vi "Result Response.vi"(8 "error in (no error)":errorcluster, 10 "Acquired Result.lvclass":refnum<class "Acquired Result.lvclass">, 11 "Measure Controller in":refnum<class "Measure Controller.lvclass">) -> (0 "error out":errorcluster, 3 "Measure Controller out":refnum<class "Measure Controller.lvclass">)   [LabVIEW 2015, in "Measure Controller.lvclass"]
uses:
  Measure Controller.lvclass
  Results/Acquired Result/Acquired Result.lvclass
  Measure Object/Measure Object.lvclass/Measure Object.ctl
  Measure Object/Read tdms stream.vi
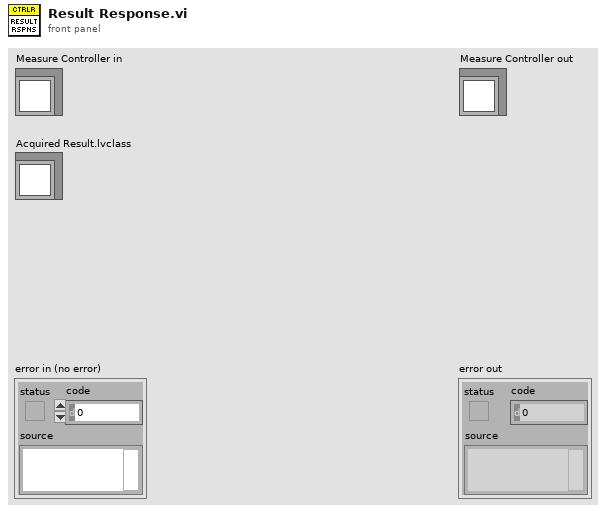
[diagram p1: front panel]
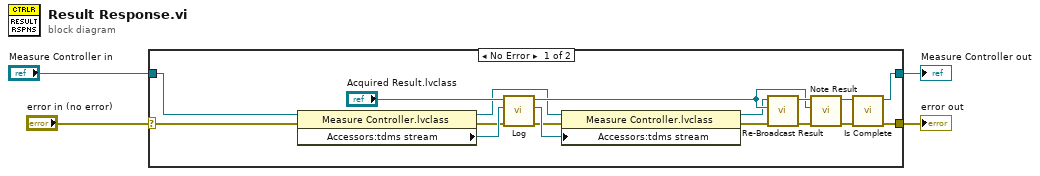
[diagram p0: block diagram]
diagram:
  n1 = case shown="No Error" "error in (no error)" {
    selector: "error in (no error)" -> [w10 w23]
    tunnel: [w20 w23] -> w3
    tunnel: [w21 w22] -> w1
    tunnel: "Measure Controller in" -> [w17 w22]
    frame No Error {
      n2 = property class="Measure Controller.lvclass"(reference=w17, error in=w10) -> (reference out=w7:refnum<class "Measure Controller.lvclass">, error out=w9:errorcluster, "Accessors:tdms stream"=w12:refnum<k34>)
      n3 = call-dynamic "Log.vi"("error in (no error)"=w9, "tdms file"=w12, "Acquired Result in"="Acquired Result.lvclass") -> ("error out"=w8:errorcluster, "tdms file out"=w11:refnum<k34>, "Acquired Result out"=w13:refnum<class "Acquired Result.lvclass">)  [unwired: 6 in]
      n4 = property class="Measure Controller.lvclass"(reference=w7, error in=w8, "Accessors:tdms stream"=w11) -> (reference out=w6:refnum<class "Measure Controller.lvclass">, error out=w5:errorcluster)
      n5 = call-dynamic "Re-Broadcast Result.vi"("error in (no error)"=w5, "Acquired Result.lvclass"=w13, "Measure Controller in"=w6) -> ("error out"=w16:errorcluster, "Measure Controller out"=w15:refnum<class "Measure Controller.lvclass">)  [unwired: 7 in]
      n6 = call-dynamic "Note Result.vi"("error in (no error)"=w16, "Acquired Result.lvclass"=w13, "Measure Controller in"=w15) -> ("error out"=w18:errorcluster, "Measure Controller out"=w19:refnum<class "Measure Controller.lvclass">)  [unwired: 7 in]
      n7 = call-dynamic "Is Complete.vi"("error in (no error)"=w18, "Measure Controller in"=w19) -> ("error out"=w20:errorcluster, "Measure Controller out"=w21:refnum<class "Measure Controller.lvclass">)  [unwired: 8 in]
    }
    frame Error {
    }
  }
  "error out" <- w3
  "Measure Controller out" <- w1
